vi "MessageName.vi"() -> (2 "MessageName":string)   [LabVIEW 2020, in "Events.lvlib"]
uses:
  Events.lvlib
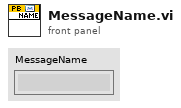
[diagram p1: front panel]
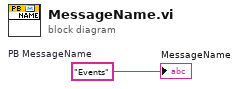
[diagram p0: block diagram]
diagram:
  w1 = "Events"  # PB MessageName
  "MessageName" <- w1
